vi "CTR_NetworkConfigs.vi"(8 "error in":errorcluster, 10 "StreamCluster_TypeDef":T1={"DAQ_Configs"=[], "CTR_Config"={"CTR refDes"="", "CTR IP Addr"=""}, "Network_Configs"={"Buffer"=1, "ManagmentRate_Hz"=1000, "StreamRate_Hz"=10, "ConnectionHysterisis"=0, "LoggingRate_Hz"=10}, "ConfigXML_Checksum"=""}, 11 "DOM document in":refnum<k20>) -> (0 "error out":errorcluster, 2 "StreamCluster_TypeDef 2":T1={"DAQ_Configs"=[], "CTR_Config"={"CTR refDes"="", "CTR IP Addr"=""}, "Network_Configs"={"Buffer"=1, "ManagmentRate_Hz"=1000, "StreamRate_Hz"=10, "ConnectionHysterisis"=0, "LoggingRate_Hz"=10}, "ConfigXML_Checksum"=""}, 3 "DOM document out":refnum<k20>)   [LabVIEW 2024]
uses:
  Control/StreamCluster_TypeDef.ctl
  Control/streamIO_states.ctl
  <vilib>/xml/Close Reference(Node).vi
  <vilib>/xml/NI_XML.lvlib
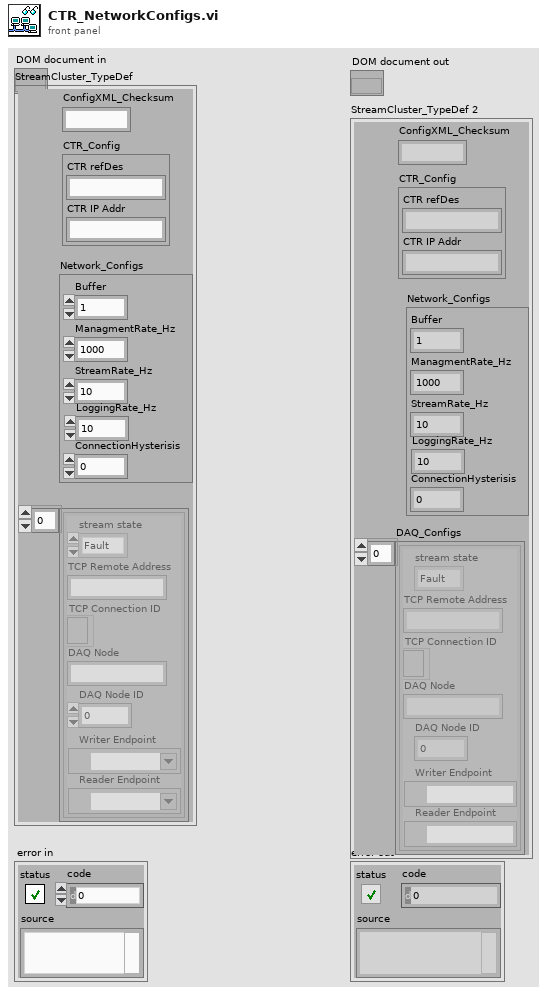
[diagram p1: front panel]
types:
  T1 = typedef "StreamCluster_TypeDef.ctl" = cluster{"DAQ_Configs":cluster{"stream state":T2, "TCP Remote Address":string, "TCP Connection ID":refnum<k5>, "DAQ Node":string, "DAQ Node ID":i32, "Writer Endpoint":refnum<k21>, "Reader Endpoint":refnum<k21>}[], "CTR_Config":cluster{"CTR refDes":string, "CTR IP Addr":string}, "Network_Configs":cluster{"Buffer":i32, "ManagmentRate_Hz":i32, "StreamRate_Hz":i32, "ConnectionHysterisis":i32, "LoggingRate_Hz":i32}, "ConfigXML_Checksum":string}
  T2 = typedef "streamIO_states.ctl" = enum16{"Fault", "Initialize", "Stream", "Close"}
  T3 = cluster{"[0]":string, "[1]":string, "[2]":string, "[3]":string, "[4]":string, "[5]":string, "[6]":string, "[7]":string, "[8]":string}
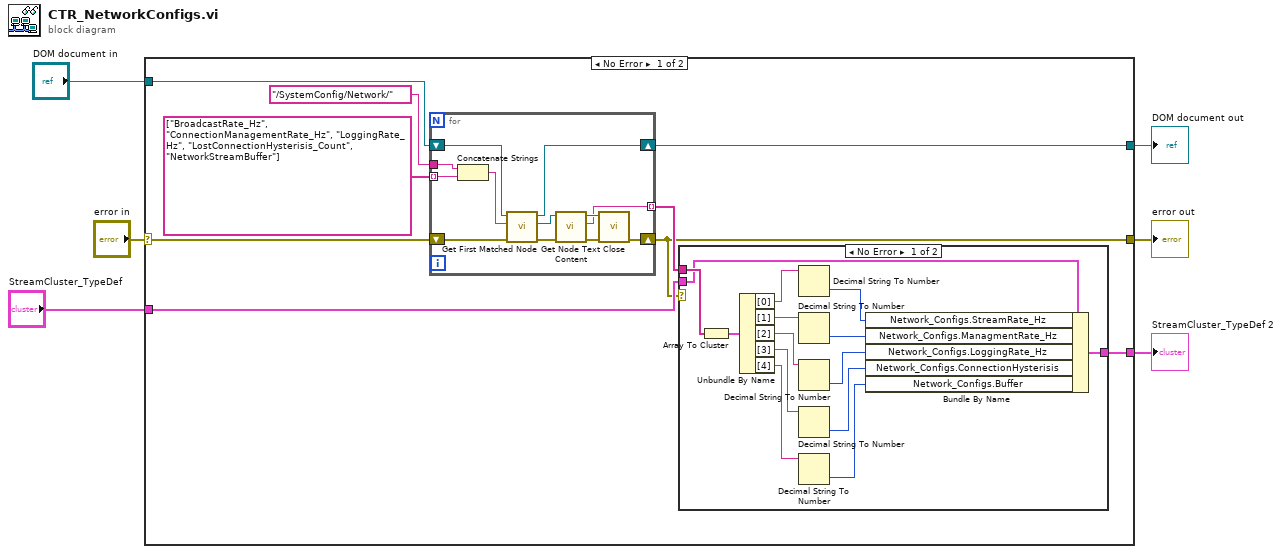
[diagram p0: block diagram]
diagram:
  n1 = case shown="No Error" "error in" {
    selector: "error in" -> [w13 w45]
    tunnel: [w7 w45] -> w5
    tunnel: "DOM document in" -> [w12 w44]
    tunnel: [w11 w44] -> w3
    tunnel: [w8 w43] -> w2
    tunnel: "StreamCluster_TypeDef" -> [w9 w43]
    frame No Error {
      n2 = for {
        tunnel: "/SystemConfig/Network/" ("XPath expression") -> [w38]
        tunnel: string[] ["BroadcastRate_Hz", "ConnectionManagementRate_Hz", "LoggingRate_Hz", "LostConnectionHysterisis_Count", "NetworkStreamBuffer"] -> [w37] mode=indexing
        shift-right: [w33] -> w11
        shift-left: w12 -> [w39]
        shift-right: [w32] -> w7
        shift-left: w13 -> [w40]
        tunnel: [w31] -> w10 mode=indexing
        n3 = Concatenate Strings(w38, w37) -> (w36:string)
        n4 = call <vilib>:"Get First Matched Node.vi"("error in (no error)"=w40, "XPath expression"=w36, "node in"=w39) -> ("error out"=w41:errorcluster, "node result"=w42:refnum<k20>, "node out"=w33:refnum<k20>)  [unwired: 6 in]
        n5 = call <vilib>:"Get Node Text Content.vi"("error in (no error)"=w41, "node in"=w42) -> ("error out"=w35:errorcluster, "node text"=w31:string, "node out"=w34:refnum<k20>)  [unwired: 7 in]
        n6 = call-poly <vilib>:"Close.vi"("error in (no error)"=w35, "node"=w34) -> ("error out"=w32:errorcluster)  [unwired: 7 out]
      }
      n7 = case shown="No Error" w7 {
        tunnel: w10 -> [w29 _]
        tunnel: w9 -> [w27 w30]
        tunnel: [w26 w30] -> w8
        frame No Error {
          n8 = Array To Cluster(array=w29) -> (cluster=w28:T3)
          n9 = Unbundle By Name(w28) -> ("[0]"=w25:string, "[1]"=w22:string, "[2]"=w20:string, "[3]"=w19:string, "[4]"=w17:string)
          n10 = Decimal String To Number(string=w25) -> (number=w24:i32)  [unwired: 2 in, 1 out]
          n11 = Decimal String To Number(string=w22) -> (number=w23:i32)  [unwired: 2 in, 1 out]
          n12 = Decimal String To Number(string=w20) -> (number=w21:i32)  [unwired: 2 in, 1 out]
          n13 = Decimal String To Number(string=w19) -> (number=w18:i32)  [unwired: 2 in, 1 out]
          n14 = Decimal String To Number(string=w17) -> (number=w16:i32)  [unwired: 2 in, 1 out]
          n15 = Bundle By Name(cluster=w27, "Network_Configs.StreamRate_Hz"=w24, "Network_Configs.ManagmentRate_Hz"=w23, "Network_Configs.LoggingRate_Hz"=w21, "Network_Configs.ConnectionHysterisis"=w18, "Network_Configs.Buffer"=w16) -> (w26:T1)
        }
        frame Error {
        }
      }
    }
    frame Error {
    }
  }
  "error out" <- w5
  "DOM document out" <- w3
  "StreamCluster_TypeDef 2" <- w2
